vi "Get All Enqueuers.vi"(8 "error in (no error)":errorcluster, 11 "Enqueuer Look Up Table in":refnum<class "Enqueuer Look Up Table.lvclass">) -> (0 "error out":errorcluster, 1 "Names":string[](array[string]), 2 "Enqueuers":refnum<class "Message Enqueuer.lvclass">[](array[class]), 3 "Enqueuer Look Up Table out":refnum<class "Enqueuer Look Up Table.lvclass">)   [LabVIEW 2016, in "Stream Mediator.lvlib" / "Enqueuer Look Up Table.lvclass"]
doc: "--\nCopyright © 2017 Composed SystemsI All rights reserved.\n\nAuthor: Jon McBee <jon.mcbee@composed.io>\n\nThis library is provided \"AS IS\" ,WITHOUT WARRANTIES OR\nCONDITIONS OF ANY KIND, either express or implied.\n\nComposed Systems -- composed.io\n\nStream 0.0.1.1\nJon McBee - Composed Systems\nCopyright (c) 2017, Composed Systems"
uses:
  <userlib>/Composed Systems/Stream/Mediator/Classes/Enqueuer Look Up Table/Enqueuer Look Up Table.lvclass
  C:/Program Files (x86)/National Instruments/LabVIEW 2016/user.lib/Composed Systems/Stream/Look Up Table/Look Up Table/Look Up Table.lvclass
  <vilib>/ActorFramework/Message Enqueuer/Message Enqueuer.lvclass
  <userlib>/Composed Systems/Stream/Look Up Table/Look Up Table/Look Up Table.lvclass
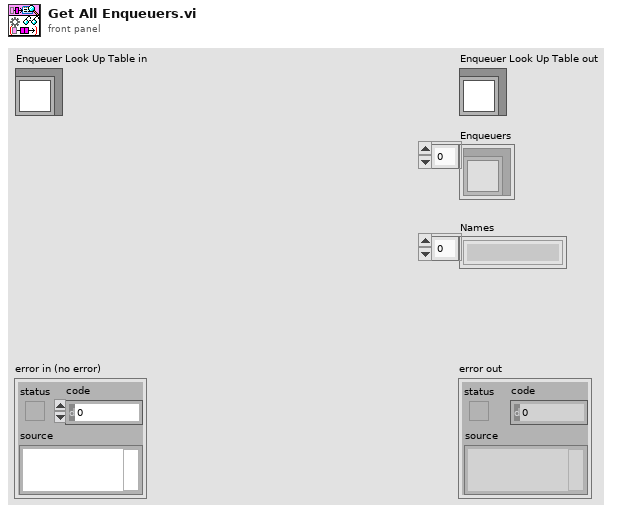
[diagram p1: front panel]
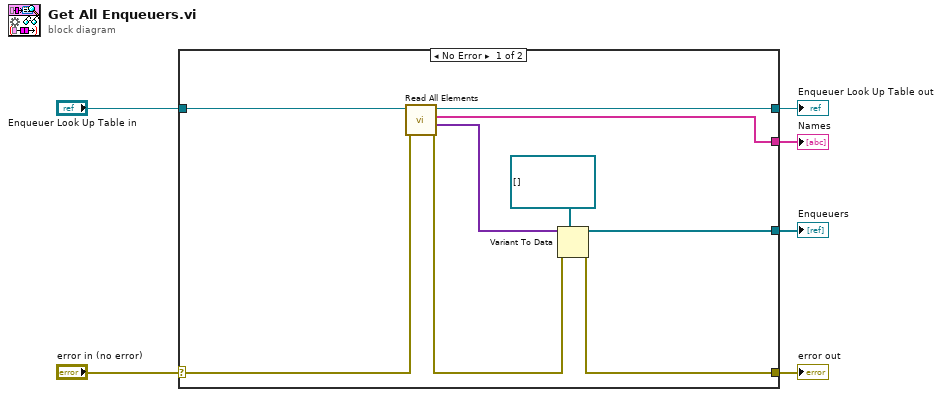
[diagram p0: block diagram]
diagram:
  n1 = case shown="No Error" "error in (no error)" {
    selector: "error in (no error)" -> [w12 w17]
    tunnel: [w15 w17] -> w5
    tunnel: [w9 w16] -> w3
    tunnel: "Enqueuer Look Up Table in" -> [w10 w16]
    tunnel: [w13 _] -> w2
    tunnel: [w8 _] -> w1
    frame No Error {
      n2 = call <userlib>:"Read All Elements.vi"("error in (no error)"=w12, "Look Up Table in"=w10) -> ("error out"=w11:errorcluster, "All Elements"=w7:variant[], "Names"=w8:string[], "Look Up Table out"=w9:refnum<class "Enqueuer Look Up Table.lvclass">)  [unwired: 6 in]
      n3 = Variant To Data(error in=w11, type=refnum<class "Message Enqueuer.lvclass">[] [], Variant=w7) -> (data=w13:refnum<class "Message Enqueuer.lvclass">[], error out=w15:errorcluster)
    }
    frame Error {
    }
  }
  "error out" <- w5
  "Enqueuer Look Up Table out" <- w3
  "Enqueuers" <- w2
  "Names" <- w1
